vi "RIODetermineChangeToTiming.vi"(8 "First Trigger Time":dbl, 9 "End Time":dbl, 10 "Start Time":dbl, 11 "Rate":dbl) -> (0 "delay_cycles":dbl, 1 "end_time":dbl, 2 "start_time":dbl, 3 "samples":dbl)   [LabVIEW 2015]
doc: "Determine the delay_cycles the RIOs shoudl wait after the PXI_Star trigger is received in order to start aquiring at the correct time.\nAlso determine the number of samples needed to aquire for the complete interval between start and end time. If necessary adjust the start and end time to fit in 20 ns increments."
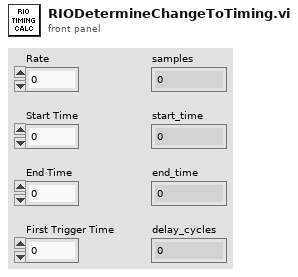
[diagram p1: front panel]
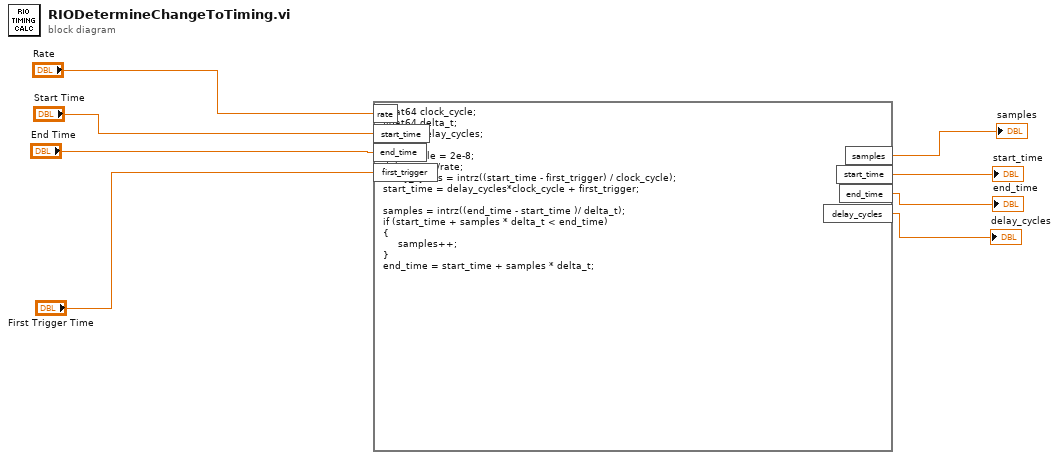
[diagram p0: block diagram]
diagram:
  n1 = formula code="float64 clock_cycle;\nfloat64 delta_t;\nfloat64 delay_cycles;\n\nclock_cycle = 2e-8;\ndelta_t = 1/rate;\ndelay_cycles = intrz((start_time - first_trigger) / clock_cycle);\nstart_time = delay_cycles*clock_cycle + first_trigger;\n\nsamples = intrz((end_time - start_time )/ delta_t);\nif (start_time + samples * delta_t < end_time)\n{\n     samples++;\n}\nend_time = start_time + samples * delta_t;"("first_trigger"="First Trigger Time", "start_time"="Start Time", "rate"="Rate", "end_time"="End Time") -> ("end_time"=→"end_time":dbl, "start_time"=→"start_time":dbl, "delay_cycles"=→"delay_cycles":dbl, "samples"=→"samples":dbl)
